vi "UDPsender_v1.vi"(11 "nums2send":dbl[](array[numeric])=[0.0, 0.0, 0.0, 0.0]) -> (3 "string2send":string)   [LabVIEW 2016]
panel:
  # "x actual [mm]"
  # "y actual [mm]"
  # "z actual [mm]"
  # "theta_1 actual [deg]"
  # ">>>"
  # "theta_2 actual [deg]"
  # "d_3 actual [mm]"
  # "theta_4 actual [deg]"
  # "q_5 []"
  # "OCTz actual [mm]"
  # "Xstage acct [mm]"
  # "Ystage acct [mm]"
  # "Zstage acct [mm]"
  # "vac cmd"
  # "hydration [0,1]"
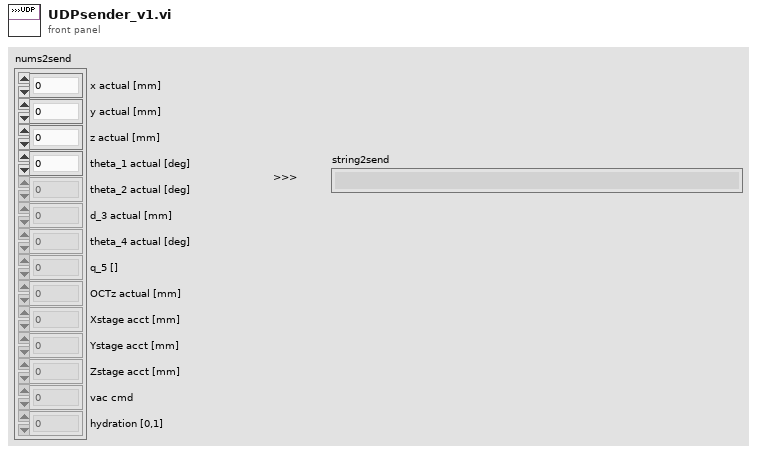
[diagram p1: front panel]
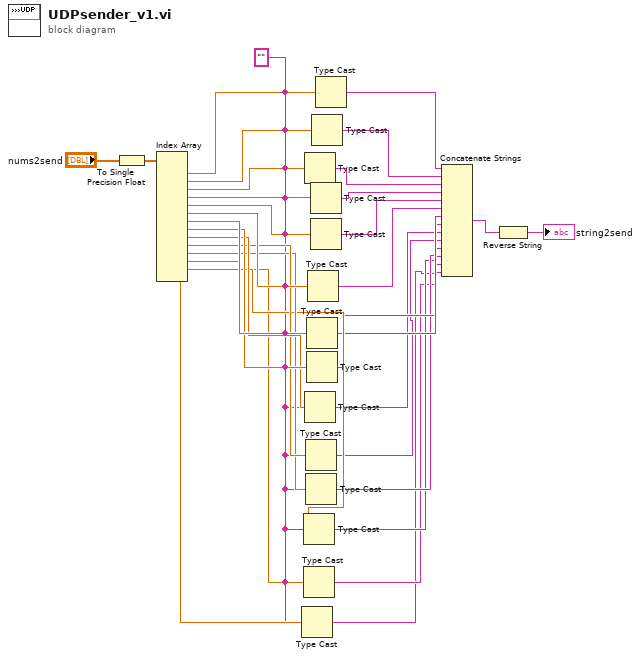
[diagram p0: block diagram]
diagram:
  w4 = "" ("data in")
  n1 = To Single Precision Float(number="nums2send") -> (single precision float=w25:sgl[])
  n2 = Index Array(array=w25) -> (element #1=w7:sgl, element #2=w6:sgl, element #3=w5:sgl, element #4=w26:sgl, element #5=w27:sgl, element #6=w28:sgl, element #7=w23:sgl, element #8=w22:sgl, element #9=w21:sgl, element #10=w20:sgl, element #11=w19:sgl, element #12=w18:sgl, element #13=w17:sgl, element #14=w16:sgl)  [unwired: 14 in]
  n3 = Type Cast(type=w4, x=w16) -> (*(type *) &x=w8:string)
  n4 = Type Cast(type=w4, x=w18) -> (*(type *) &x=w10:string)
  n5 = Type Cast(type=w4, x=w17) -> (*(type *) &x=w9:string)
  n6 = Type Cast(type=w4, x=w5) -> (*(type *) &x=w1:string)
  n7 = Type Cast(type=w4, x=w21) -> (*(type *) &x=w13:string)
  n8 = Type Cast(type=w4, x=w20) -> (*(type *) &x=w12:string)
  n9 = Type Cast(type=w4, x=w19) -> (*(type *) &x=w11:string)
  n10 = Type Cast(type=w4, x=w23) -> (*(type *) &x=w15:string)
  n11 = Type Cast(type=w4, x=w22) -> (*(type *) &x=w14:string)
  n12 = Type Cast(type=w4, x=w28) -> (*(type *) &x=w30:string)
  n13 = Type Cast(type=w4, x=w26) -> (*(type *) &x=w32:string)
  n14 = Type Cast(type=w4, x=w27) -> (*(type *) &x=w29:string)
  n15 = Type Cast(type=w4, x=w6) -> (*(type *) &x=w2:string)
  n16 = Type Cast(type=w4, x=w7) -> (*(type *) &x=w3:string)
  n17 = Concatenate Strings(w3, w2, w1, w32, w29, w30, w15, w14, w13, w12, w11, w10, w9, w8) -> (w31:string)
  n18 = Reverse String(1:w31) -> (0:→"string2send":string)
